vi "IB_RW_Project_Source_File.vi"(7 "action":T3, 8 "error in (no error)":errorcluster, 9 "index in":string, 10 "file in":T2, 11 "buildObject":T1) -> (0 "error out":errorcluster, 1 "index out":string, 2 "file out":T2, 3 "buildObject out":T1)   [LabVIEW 2020]
doc: "Reads and writes the data to the object property bag."
uses:
  <resource>/Framework/Providers/API/ItemRef.ctl
  <vilib>/AppBuilder/IB_RW_Project/IB_RW_Project_Source_File_Data.ctl
  <vilib>/AppBuilder/IB_RW_Project/IB_RW_Project_PropBag_Action.ctl
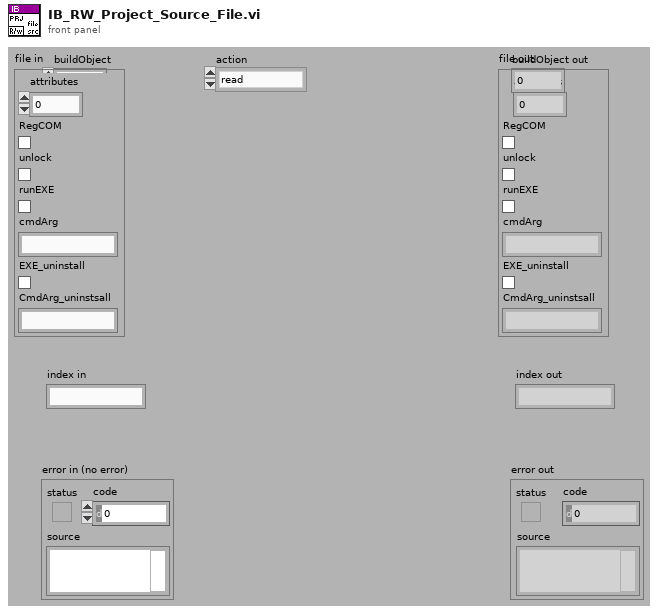
[diagram p1: front panel]
types:
  T1 = typedef "ItemRef.ctl" = u64
  T2 = typedef "IB_RW_Project_Source_File_Data.ctl" = cluster{"attributes":i16, "RegCOM":bool, "unlock":bool, "runEXE":bool, "cmdArg":string, "EXE_uninstall":bool, "CmdArg_uninstsall":string}
  T3 = typedef "IB_RW_Project_PropBag_Action.ctl" = enum16{"read", "write", "clear", "readPrevious", "writePrevious", "clearPrevious"}
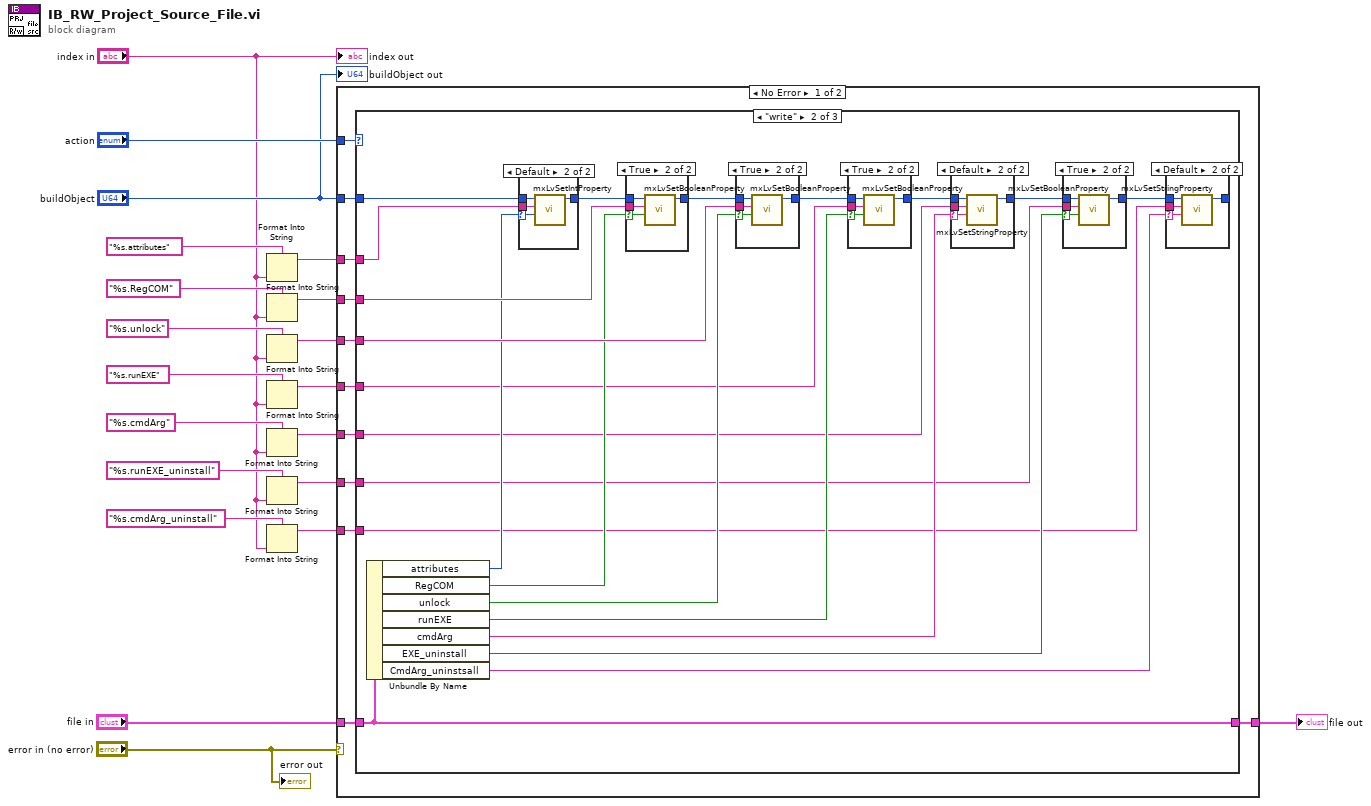
[diagram p0: block diagram]
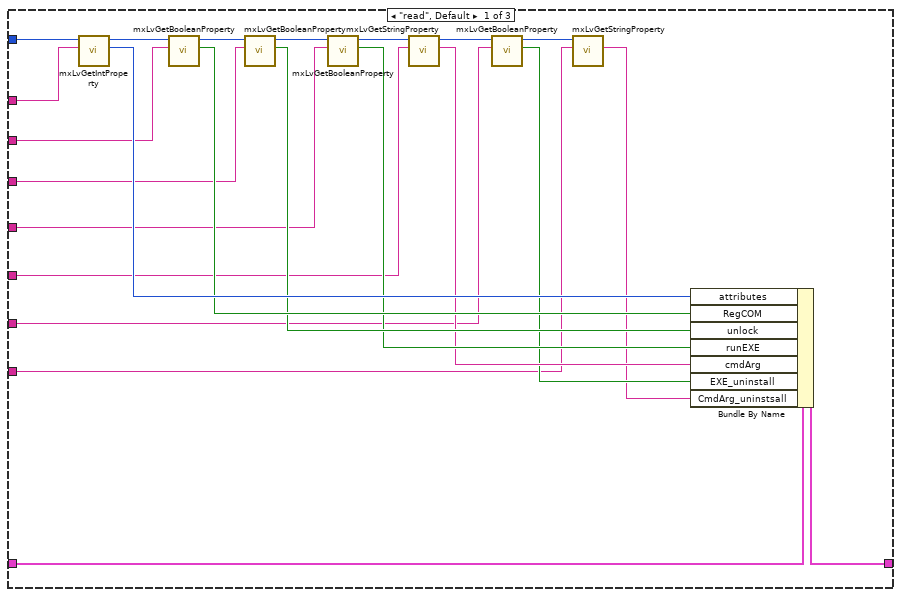
[diagram p2: hidden frame]
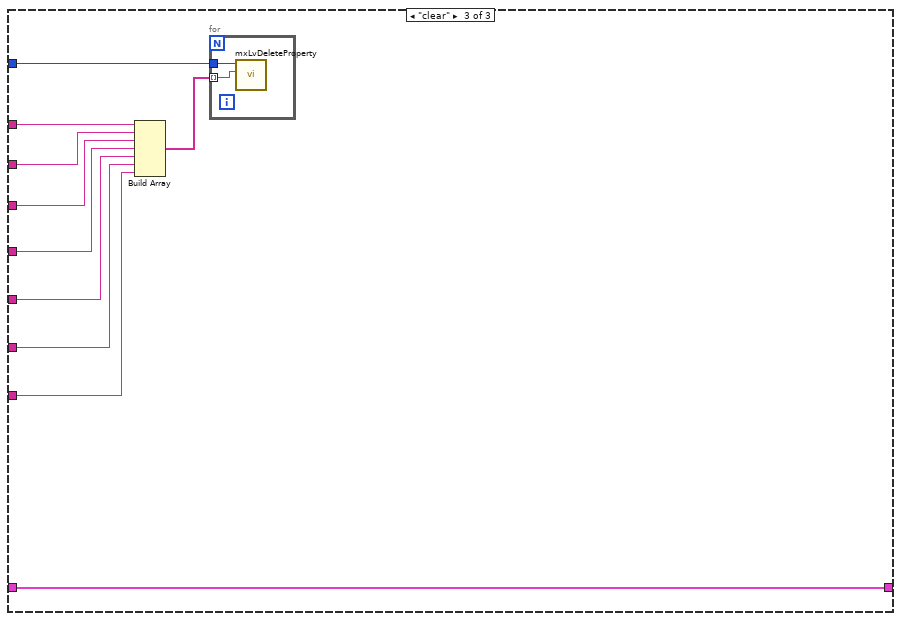
[diagram p10: hidden frame]
diagram:
  n1 = Format Into String(format string="%s.attributes", "index in") -> (resulting string=w12:string)  [unwired: 2 in, 1 out]
  n2 = Format Into String(format string="%s.RegCOM", "index in") -> (resulting string=w11:string)  [unwired: 2 in, 1 out]
  n3 = Format Into String(format string="%s.unlock", "index in") -> (resulting string=w10:string)  [unwired: 2 in, 1 out]
  n4 = Format Into String(format string="%s.runEXE", "index in") -> (resulting string=w8:string)  [unwired: 2 in, 1 out]
  n5 = Format Into String(format string="%s.cmdArg", "index in") -> (resulting string=w6:string)  [unwired: 2 in, 1 out]
  n6 = Format Into String(format string="%s.runEXE_uninstall", "index in") -> (resulting string=w2:string)  [unwired: 2 in, 1 out]
  n7 = Format Into String(format string="%s.cmdArg_uninstall", "index in") -> (resulting string=w1:string)  [unwired: 2 in, 1 out]
  n8 = case shown="No Error" "error in (no error)" {
    tunnel: "action" -> [w31 _]
    tunnel: "file in" -> [w30 w124]
    tunnel: [w29 w124] -> w18
    tunnel: "buildObject" -> [w28 _]
    tunnel: w12 -> [w27 _]
    tunnel: w11 -> [w26 _]
    tunnel: w10 -> [w25 _]
    tunnel: w8 -> [w24 _]
    tunnel: w6 -> [w23 _]
    tunnel: w2 -> [w22 _]
    tunnel: w1 -> [w21 _]
    frame No Error {
      n9 = case shown="\"write\"" w31 {
        tunnel: w28 -> [w54 w75 w116]
        tunnel: w30 -> [w52 w76 w121]
        tunnel: [w51 w76 w121] -> w29
        tunnel: w27 -> [w53 w74 w119]
        tunnel: w26 -> [w48 w71 w118]
        tunnel: w25 -> [w45 w70 w117]
        tunnel: w24 -> [w41 w65 w115]
        tunnel: w23 -> [w38 w63 w114]
        tunnel: w22 -> [w33 w56 w113]
        tunnel: w21 -> [w32 w55 w112]
        frame "read", Default {
          n10 = call <resource>:"mxLvGetIntProperty.vi"("Tag"=w53, "Item"=w54) -> ("Value"=w50:i32, "Item"=w49:T1)  [unwired: 1 in, 7 out]
          n11 = call <resource>:"mxLvGetBooleanProperty.vi"("Tag"=w48, "Item"=w49) -> ("Value"=w47:bool, "Item"=w46:T1)  [unwired: 1 in, 7 out]
          n12 = call <resource>:"mxLvGetBooleanProperty.vi"("Tag"=w45, "Item"=w46) -> ("Value"=w44:bool, "Item"=w43:T1)  [unwired: 1 in, 7 out]
          n13 = call <resource>:"mxLvGetBooleanProperty.vi"("Tag"=w41, "Item"=w43) -> ("Value"=w42:bool, "Item"=w40:T1)  [unwired: 1 in, 7 out]
          n14 = call <resource>:"mxLvGetStringProperty.vi"("Tag"=w38, "Item"=w40) -> ("Value"=w39:string, "Item"=w36:T1)  [unwired: 1 in, 7 out]
          n15 = call <resource>:"mxLvGetBooleanProperty.vi"("Tag"=w33, "Item"=w36) -> ("Value"=w35:bool, "Item"=w37:T1)  [unwired: 1 in, 7 out]
          n16 = call <resource>:"mxLvGetStringProperty.vi"("Tag"=w32, "Item"=w37) -> ("Value"=w34:string)  [unwired: 1 in, 8 out]
          n17 = Bundle By Name(cluster=w52, "attributes"=w50, "RegCOM"=w47, "unlock"=w44, "runEXE"=w42, "cmdArg"=w39, "EXE_uninstall"=w35, "CmdArg_uninstsall"=w34) -> (w51:T2)
        }
        frame "write" {
          n18 = Unbundle By Name(w76) -> ("attributes"=w69:i16, "RegCOM"=w68:bool, "unlock"=w67:bool, "runEXE"=w66:bool, "cmdArg"=w61:string, "EXE_uninstall"=w58:bool, "CmdArg_uninstsall"=w57:string)
          n19 = case shown="Default" w69 {
            selector: w69 -> [_ w108]
            tunnel: w75 -> [w107 w111]
            tunnel: w74 -> [_ w110]
            tunnel: [w107 w109] -> w73
            frame 0 {
            }
            frame Default {
              n20 = call <resource>:"mxLvSetIntProperty.vi"("Value (0)"=w108, "Tag"=w110, "Item"=w111) -> ("Item"=w109:T1)  [unwired: 2 in, 6 out]
            }
          }
          n21 = case shown="True" w68 {
            selector: w68 -> [_ w103]
            tunnel: w73 -> [w102 w106]
            tunnel: [w102 w105] -> w72
            tunnel: w71 -> [_ w104]
            frame False {
            }
            frame True {
              n22 = call <resource>:"mxLvSetBooleanProperty.vi"("Value (F)"=w103, "Tag"=w104, "Item"=w106) -> ("Item"=w105:T1)  [unwired: 2 in, 6 out]
            }
          }
          n23 = case shown="True" w67 {
            selector: w67 -> [_ w99]
            tunnel: w72 -> [w97 w101]
            tunnel: w70 -> [_ w100]
            tunnel: [w97 w98] -> w64
            frame False {
            }
            frame True {
              n24 = call <resource>:"mxLvSetBooleanProperty.vi"("Value (F)"=w99, "Tag"=w100, "Item"=w101) -> ("Item"=w98:T1)  [unwired: 2 in, 6 out]
            }
          }
          n25 = case shown="True" w66 {
            selector: w66 -> [_ w94]
            tunnel: w64 -> [w92 w96]
            tunnel: w65 -> [_ w95]
            tunnel: [w92 w93] -> w62
            frame False {
            }
            frame True {
              n26 = call <resource>:"mxLvSetBooleanProperty.vi"("Value (F)"=w94, "Tag"=w95, "Item"=w96) -> ("Item"=w93:T1)  [unwired: 2 in, 6 out]
            }
          }
          n27 = case shown="Default" w61 {
            selector: w61 -> [_ w88]
            tunnel: w62 -> [w87 w91]
            tunnel: w63 -> [_ w90]
            tunnel: [w87 w89] -> w59
            frame "" {
            }
            frame Default {
              n28 = call <resource>:"mxLvSetStringProperty.vi"("Value (\"\")"=w88, "Tag"=w90, "Item"=w91) -> ("Item"=w89:T1)  [unwired: 2 in, 6 out]
            }
          }
          n29 = case shown="True" w58 {
            selector: w58 -> [_ w84]
            tunnel: w59 -> [w82 w86]
            tunnel: w56 -> [_ w85]
            tunnel: [w82 w83] -> w60
            frame False {
            }
            frame True {
              n30 = call <resource>:"mxLvSetBooleanProperty.vi"("Value (F)"=w84, "Tag"=w85, "Item"=w86) -> ("Item"=w83:T1)  [unwired: 2 in, 6 out]
            }
          }
          n31 = case shown="Default" w57 {
            selector: w57 -> [_ w78]
            tunnel: w60 -> [w77 w81]
            tunnel: w55 -> [_ w80]
            tunnel: [w77 w79] -> _
            frame "" {
            }
            frame Default {
              n32 = call <resource>:"mxLvSetStringProperty.vi"("Value (\"\")"=w78, "Tag"=w80, "Item"=w81) -> ("Item"=w79:T1)  [unwired: 2 in, 6 out]
            }
          }
        }
        frame "clear" {
          n33 = Build Array(w119, w118, w117, w115, w114, w113, w112) -> (w120:string[])
          n34 = for {
            tunnel: w120 -> [w123] mode=indexing
            tunnel: w116 -> [w122]
            n35 = call <resource>:"mxLvDeleteProperty.vi"("Tag"=w123, "Item"=w122) -> ()  [unwired: 1 in, 9 out]
          }
        }
      }
    }
    frame Error {
    }
  }
  "file out" <- w18
  "error out" <- "error in (no error)"
  "buildObject out" <- "buildObject"
  "index out" <- "index in"
